vi "Translator.FormatEnumSrc.vi"(0 "text in":string, 1 "quotas?(T)":bool=TRUE) -> (2 "text out":string)   [LabVIEW 2016]
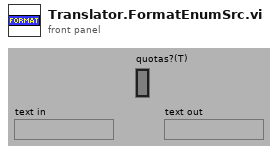
[diagram p1: front panel]
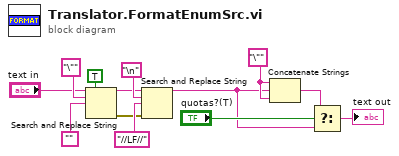
[diagram p0: block diagram]
diagram:
  w7 = "\""
  n1 = Search and Replace String(replace all?=TRUE ("replace all? (F)"), input string="text in", search string="\"", replace string="") -> (result string=w5:string, error out=w6:errorcluster)  [unwired: 4 in, 2 out]
  n2 = Search and Replace String(input string=w5, search string="\n", replace string="//LF//" ("search string"), error in=w6) -> (result string=w2:string)  [unwired: 1 in, 6 out]
  n3 = Concatenate Strings(w7, w2, w7) -> (w3:string)
  n4 = Select(t=w3, s="quotas?(T)", f=w2) -> (s? t:f=→"text out":string)
